vi "AIT 1553 - Read Parameters.vi"(0 "File Path":path, 5 "Bus In":T1, 11 "error in (no error)":errorcluster) -> (6 "Bus Out":T1, 15 "error out":errorcluster)   [LabVIEW 2013, in "AIT 1553 Custom Device.lvlib"]
uses:
  AIT 1553 Custom Device.lvlib
  Controls/1553_Bus.ctl
  Controls/1553_Bus_Controller.ctl
  Controls/1553_BC_Message.ctl
  Controls/1553 Param.ctl
  Controls/1553_Acyclic_Frame.ctl
  Controls/1553_Bus_Monitor.ctl
  Controls/1553_BM_Message.ctl
  Controls/1553_RT_Message.ctl
  <vilib>/NI/GXML/GXML.lvlib
  <vilib>/NI/GXML/_subVIs/GXML SearchParser/Search Parser.vi
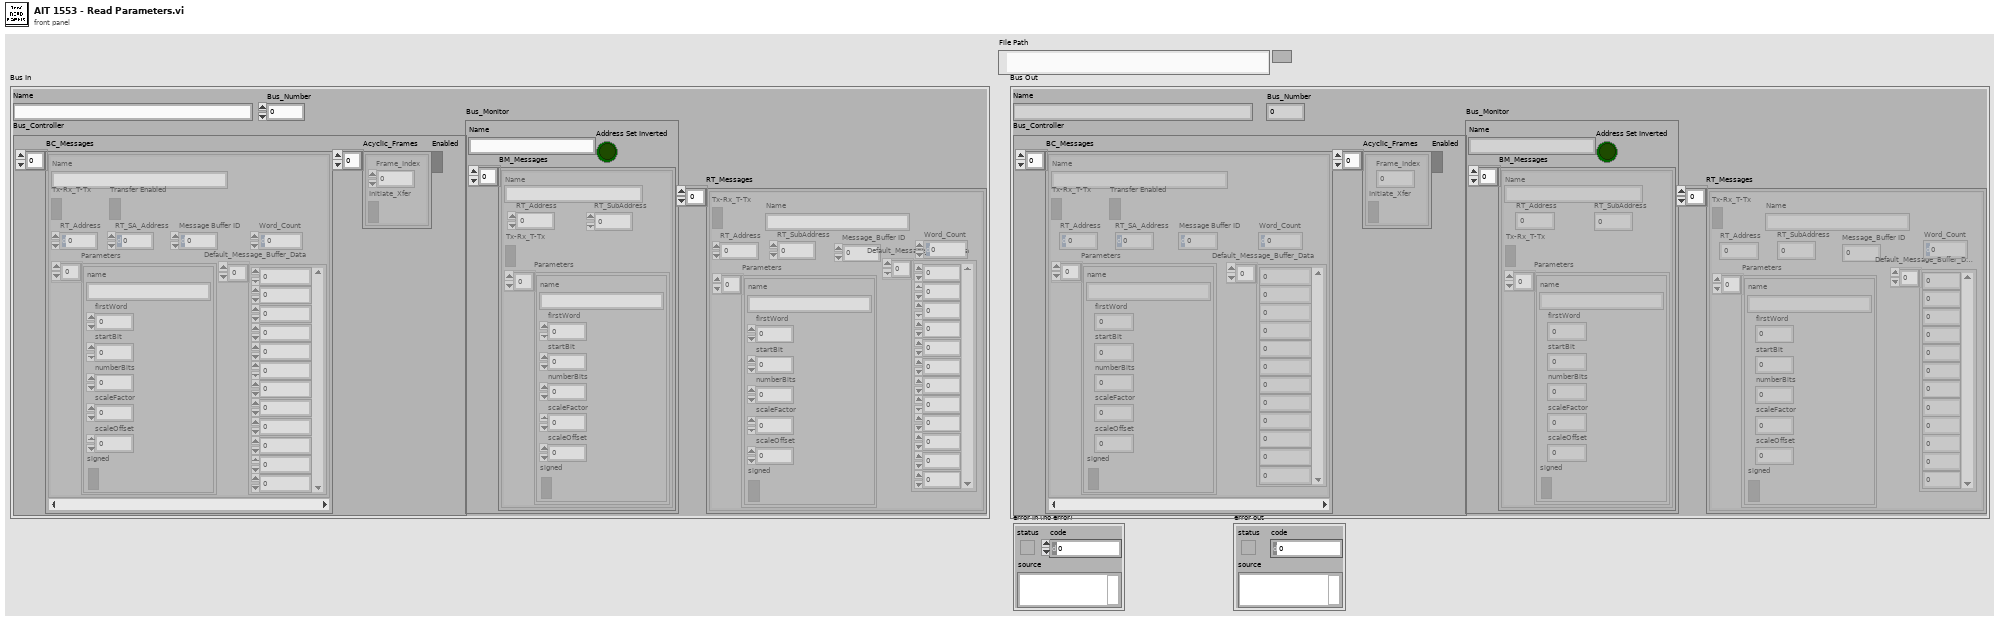
[diagram p1: front panel]
types:
  T1 = typedef "AIT 1553 Custom Device.lvlib/1553_Bus.ctl" = cluster{"Name":string, "Bus_Number":u8, "Bus_Controller":T2, "Bus_Monitor":T6, "RT_Messages":T8[]}
  T2 = typedef "AIT 1553 Custom Device.lvlib/1553_Bus_Controller.ctl" = cluster{"BC_Messages":T3[], "Acyclic_Frames":T5[], "Enabled":bool}
  T3 = typedef "AIT 1553 Custom Device.lvlib/1553_BC_Message.ctl" = cluster{"Name":string, "Tx-Rx_T-Tx":bool, "RT_Address":u8, "RT_SA_Address":u8, "Parameters":T4[], "Transfer Enabled":bool, "Message Buffer ID":u16, "Default_Message_Buffer_Data":u16[], "Word_Count":u8}
  T4 = typedef "AIT 1553 Custom Device.lvlib/1553 Param.ctl" = cluster{"name":string, "firstWord":i32, "startBit":i32, "numberBits":i32, "scaleFactor":dbl, "scaleOffset":dbl, "signed":bool}
  T5 = typedef "AIT 1553 Custom Device.lvlib/1553_Acyclic_Frame.ctl" = cluster{"Frame_Index":u8, "Initiate_Xfer":bool}
  T6 = typedef "AIT 1553 Custom Device.lvlib/1553_Bus_Monitor.ctl" = cluster{"Name":string, "BM_Messages":T7[], "Address Set Inverted":bool}
  T7 = typedef "AIT 1553 Custom Device.lvlib/1553_BM_Message.ctl" = cluster{"RT_Address":u8, "RT_SubAddress":u8, "Tx-Rx_T-Tx":bool, "Parameters":T4[], "Name":string}
  T8 = typedef "AIT 1553 Custom Device.lvlib/1553_RT_Message.ctl" = cluster{"RT_Address":u8, "RT_SubAddress":u8, "Tx-Rx_T-Tx":bool, "Parameters":T4[], "Message_Buffer ID":u16, "Default_Message_Buffer_Data":u16[], "Word_Count":u8, "Name":string}
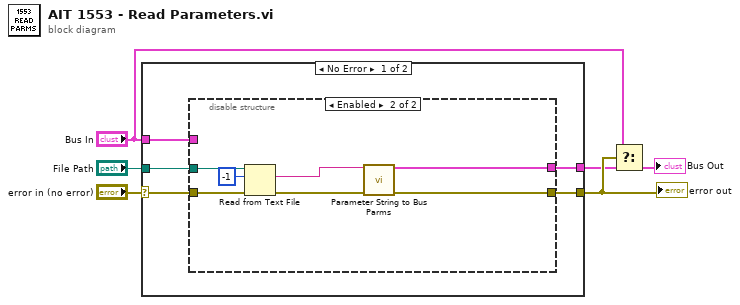
[diagram p0: block diagram]
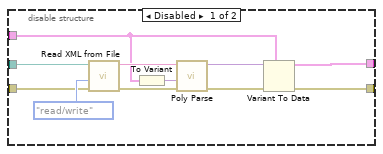
[diagram p2: hidden frame]
diagram:
  n1 = case shown="No Error" "error in (no error)" {
    selector: "error in (no error)" -> [w11 w31]
    tunnel: [w9 w31] -> w4
    tunnel: "File Path" -> [w10 _]
    tunnel: "Bus In" -> [w7 w30]
    tunnel: [w8 w30] -> w2
    frame No Error {
      n2 = disable-structure shown="Enabled" {
        disable-tunnel: w11 -> [w21 w29]
        disable-tunnel: w10 -> [w20 w28]
        disable-tunnel: [w15 w25] -> w9
        disable-tunnel: [w14 w23] -> w8
        disable-tunnel: w7 -> [w13 _]
        frame Disabled {
          n3 = call <vilib>:"Read XML from File.vi"("error in"=w21, "file access"=enum16{"read/write", "read-only", "write-only"}."read/write", "XML File Path"=w20) -> ("error out"=w17:errorcluster, "XML String Out"=w16:string)  [unwired: 7 in]
          n4 = To Variant(anything=w13) -> (Variant=w12:variant)
          n5 = call-poly <vilib>:"Poly Parse.vi"("error in"=w17, "TypeDesc"=w12, "XML String In"=w16) -> ("error out"=w18:errorcluster, "Parsed Data"=w19:variant)  [unwired: 7 in]
          n6 = Variant To Data(error in=w18, type=w13, Variant=w19) -> (data=w14:T1, error out=w15:errorcluster)
        }
        frame Enabled {
          n7 = Read from Text File(file (use dialog)=w28, count=-1, error in=w29) -> (text=w24:string, error out=w26:errorcluster)  [unwired: 1 in, 2 out]
          n8 = call "Parameter String to Bus Parms.vi"("Parms List"=w24, "error in (no error)"=w26) -> ("Bus"=w23:T1, "error out"=w25:errorcluster)  [unwired: 12 in]
        }
      }
    }
    frame Error {
    }
  }
  "error out" <- w4
  n9 = Select(t="Bus In", s=w4, f=w2) -> (s? t:f=→"Bus Out":T1)
